vi "Destroy.vi"(8 "error in (no error)":errorcluster, 11 "File Sink in":refnum<class "File Sink.lvclass">) -> (0 "error out":errorcluster)   [LabVIEW 2020, in "LV Log.lvlib" / "File Sink.lvclass"]
uses:
  File Sink.lvclass
  File Sink.lvclass/File Sink.ctl
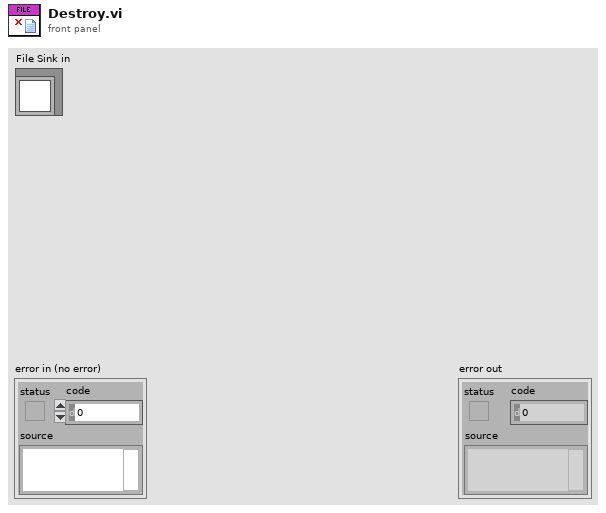
[diagram p1: front panel]
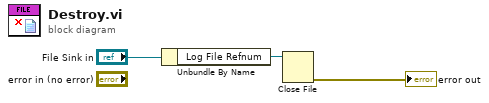
[diagram p0: block diagram]
diagram:
  n1 = Unbundle By Name("File Sink in") -> ("Log File Refnum"=w2:refnum<file>)
  n2 = Close File(refnum=w2) -> (error out=→"error out":errorcluster)  [unwired: 1 in, 1 out]
